vi "NoParent_DefaultValuesSet.vi"() -> (0 "error out":errorcluster)   [LabVIEW 2019, in "ResultTreeTest.lvlib" / "AddTestSuite.lvlib"]
uses:
  2a6c7ef5-d8ea-4de4-ba7d-c6663dbf2225.vi
  Constraint/IsEqual/Create.vi
  Constraint/IsEqual/IsEqual.lvclass
  AddTestSuite.lvlib
  ResultTree/ResultTree.lvclass
panel:
  in  "Tree":string(tree)
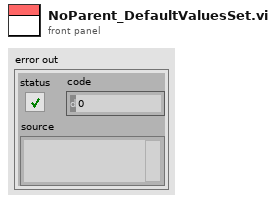
[diagram p1: front panel]
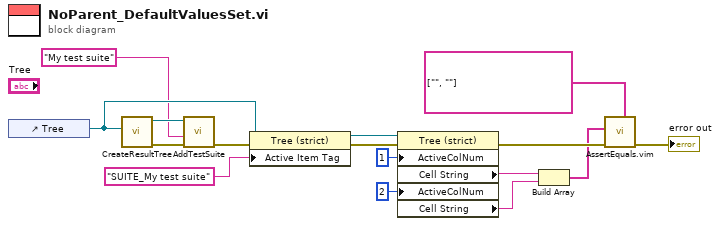
[diagram p0: block diagram]
diagram:
  n1 = control-ref of="Tree"() -> (w15:refnum<vi>)
  n2 = call "CreateResultTree.vi"("Tree Refnum"=w15) -> ("error out"=w14:errorcluster, "ResultTree out"=w12:refnum<class "ResultTree.lvclass">)  [unwired: 9 in]
  n3 = call "AddTestSuite.vi"("error in (no error)"=w14, "Name"="My test suite", "ResultTree in"=w12) -> ("error out"=w13:errorcluster)  [unwired: 6 in, 2 out]
  n4 = property class="Tree (strict)"(reference=w15, error in=w13, "Active Item Tag"="SUITE_My test suite" ("Active Item:Tag")) -> (reference out=w8:refnum<vi>, error out=w11:errorcluster)
  n5 = property class="Tree (strict)"(reference=w8, error in=w11, "ActiveColNum"=1 ("Active Cell:Active Column Number"), "ActiveColNum"=2 ("Active Cell:Active Column Number")) -> (error out=w9:errorcluster, "Cell String"=w5:string, "Cell String"=w4:string)  [unwired: 1 out]
  n6 = Build Array(w5, w4) -> (w3:string[])
  n7 = call "AssertEquals.vim"("Expected"=string[] ["", ""] ("All Tags"), "error in (no error)"=w9, "Actual"=w3) -> ("error out"=→"error out":errorcluster)  [unwired: 8 in]
